vi "LI-U8 convert U8 array number to hex string.vi"(4 "Large number -U8":T1) -> (1 "hex string (MSD 1st)":string)   [LabVIEW 2013]
doc: "Converts a large integer in U8 array format to hex string (with MSD first)."
uses:
  User Access Type defs/Large number - U8 array.ctl
panel:
  # "<<LSD"
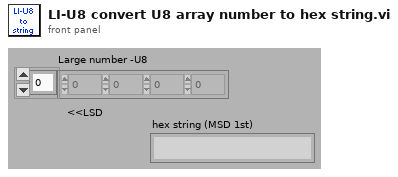
[diagram p1: front panel]
types:
  T1 = typedef "Large number - U8 array.ctl" = u8[]
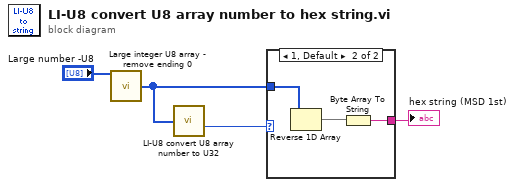
[diagram p0: block diagram]
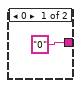
[diagram p2: hidden frame]
diagram:
  n1 = call "Large integer U8 array - remove ending 0.vi"("Large number - U8"="Large number -U8") -> ("MSD zeros removed"=w2:T1)  [unwired: 4 out]
  n2 = call "LI-U8 convert U8 array number to U32.vi"("Large number -U8"=w2) -> ("U32"=w1:u32)  [unwired: 4 out]
  n3 = case shown="1, Default" w1 {
    tunnel: w2 -> [_ w8]
    tunnel: ["0" ("string") w6] -> w3
    frame 0 {
    }
    frame 1, Default {
      n4 = Reverse 1D Array(array=w8) -> (reversed array=w7:T1)
      n5 = Byte Array To String(unsigned byte array=w7) -> (string=w6:string)
    }
  }
  "hex string (MSD 1st)" <- w3
